vi "NumToGreek.vi"(1 "Number":u8) -> (0 "Greek Letter":string)   [LabVIEW 2014]
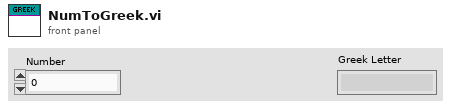
[diagram p1: front panel]
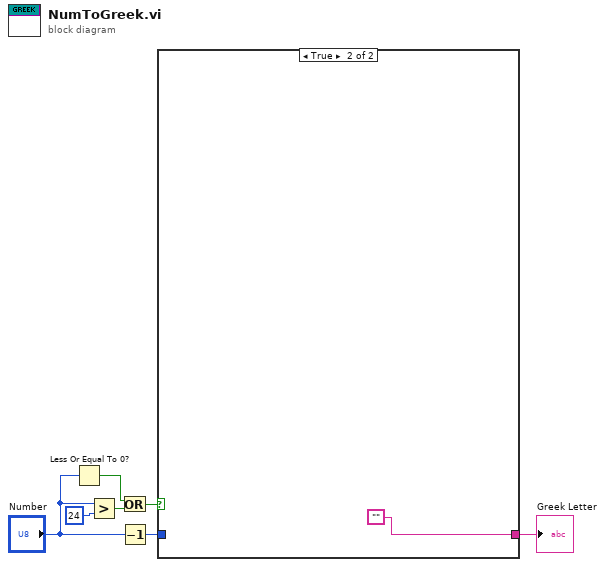
[diagram p0: block diagram]
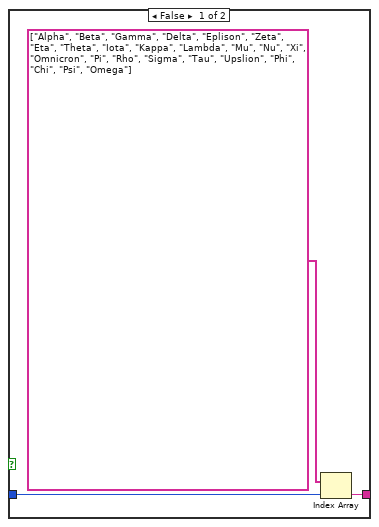
[diagram p2: hidden frame]
diagram:
  n1 = Less Or Equal To 0?(x="Number") -> (x <= 0?=w4:bool)
  n2 = Greater?(x="Number", y=24) -> (0:w5:bool)
  n3 = Or(x=w4, y=w5) -> (x .or. y?=w2:bool)
  n4 = Decrement(x="Number") -> (x-1=w1:u8)
  n5 = case shown="True" w2 {
    tunnel: [w9 ""] -> w3
    tunnel: w1 -> [w8 _]
    frame False {
      n6 = Index Array(array=string[] ["Alpha", "Beta", "Gamma", "Delta", "Eplison", "Zeta", "Eta", "Theta", "Iota", "Kappa", "Lambda", "Mu", "Nu", "Xi", "Omnicron", "Pi", "Rho", "Sigma", "Tau", "Upslion", "Phi", "Chi", "Psi", "Omega"], index=w8) -> (element=w9:string)
    }
    frame True {
    }
  }
  "Greek Letter" <- w3
